vi "Main.vi"() -> ()   [LabVIEW 2018]
doc: "This is the main VI for the application using the VICI universal electric actuator.\n\n\n(Nimble Focus Consulting 2019)"
uses:
  controls/Timing and Position Entry.ctl
  controls/Application States.ctl
  subVIs/Elapsed Timer FGV/Enum - Programme Checker Machine State Typedef.ctl
panel:
  out "Current Actuation Cycles":u32
  in  "Get Current No. of Cycles":bool
  out "Current Time (s)":u32
  out "Current Position":u32
  in  "Manual Control Tab":enum32{"Page 1"}(tab)
  in  "Set Position":bool
  in  "Decrement Position":bool
  in  "Increment Position":bool
  in  "Home":bool
  in  "Get Position":bool
  out "Current Position":u32
  in  "New Position":u32=1 min=1 max=100
  in  "Start":bool
  out "No. of entries":i32
  out "Current Entry":T1
  in  "Abort":bool
  in  "Exit":bool
  in  "Clear List":bool
  in  "Timing and Position List":T1[](array[typedef])
  in  "VISA resource name":refnum<visa-resource-name>
  # "Operation Information"
  # "For program use - do not remove."
  # "Actuator Manual Controls"
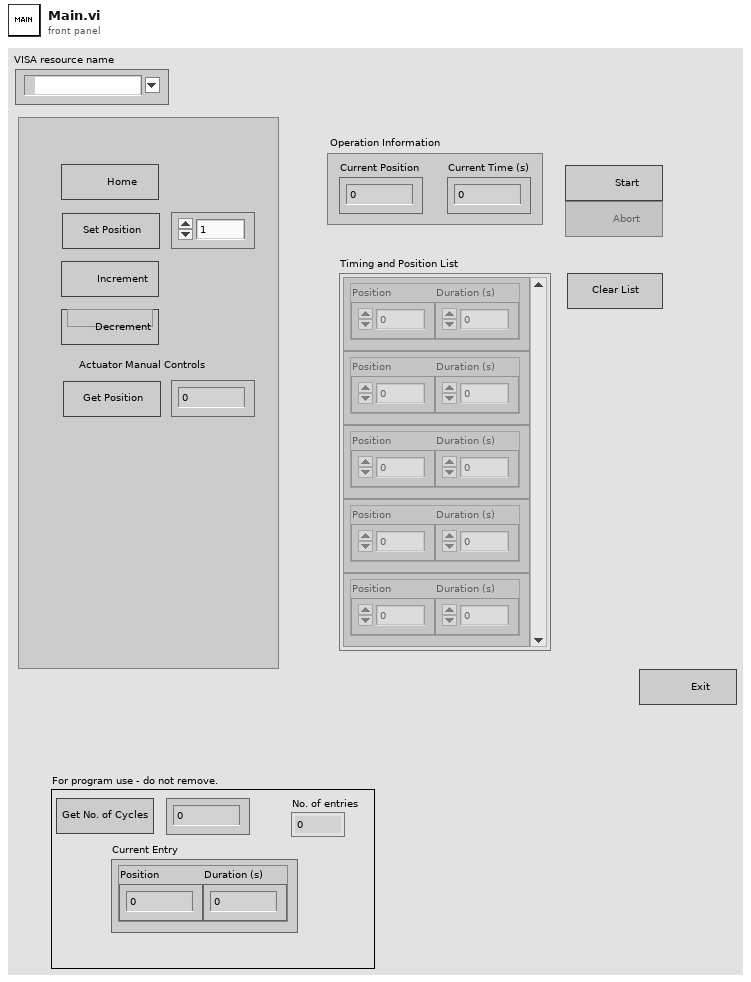
[diagram p1: front panel]
types:
  T1 = typedef "Timing and Position Entry.ctl" = cluster{"Position":u32, "Duration (s)":i32}
  T2 = typedef "Application States.ctl" = enum16{"Initialize", "Wait for Event", "Set Position", "Get Current Position", "Get Current No. of Cycles", "Home Actuator", "Increment Position", "Decrement Position", "Start Operation", "Retrieve Next Entry", "Set Position and Reset Timing", "Check Elapsed Time", "End Operation", "No More Entries Dialog", "Exit"}
  T3 = enum8{"Enabled", "Disabled", "Disabled and Grayed Out"}
  T4 = typedef "Enum - Programme Checker Machine State Typedef.ctl" = enum16{"Reset", "Check Elapsed Time"}
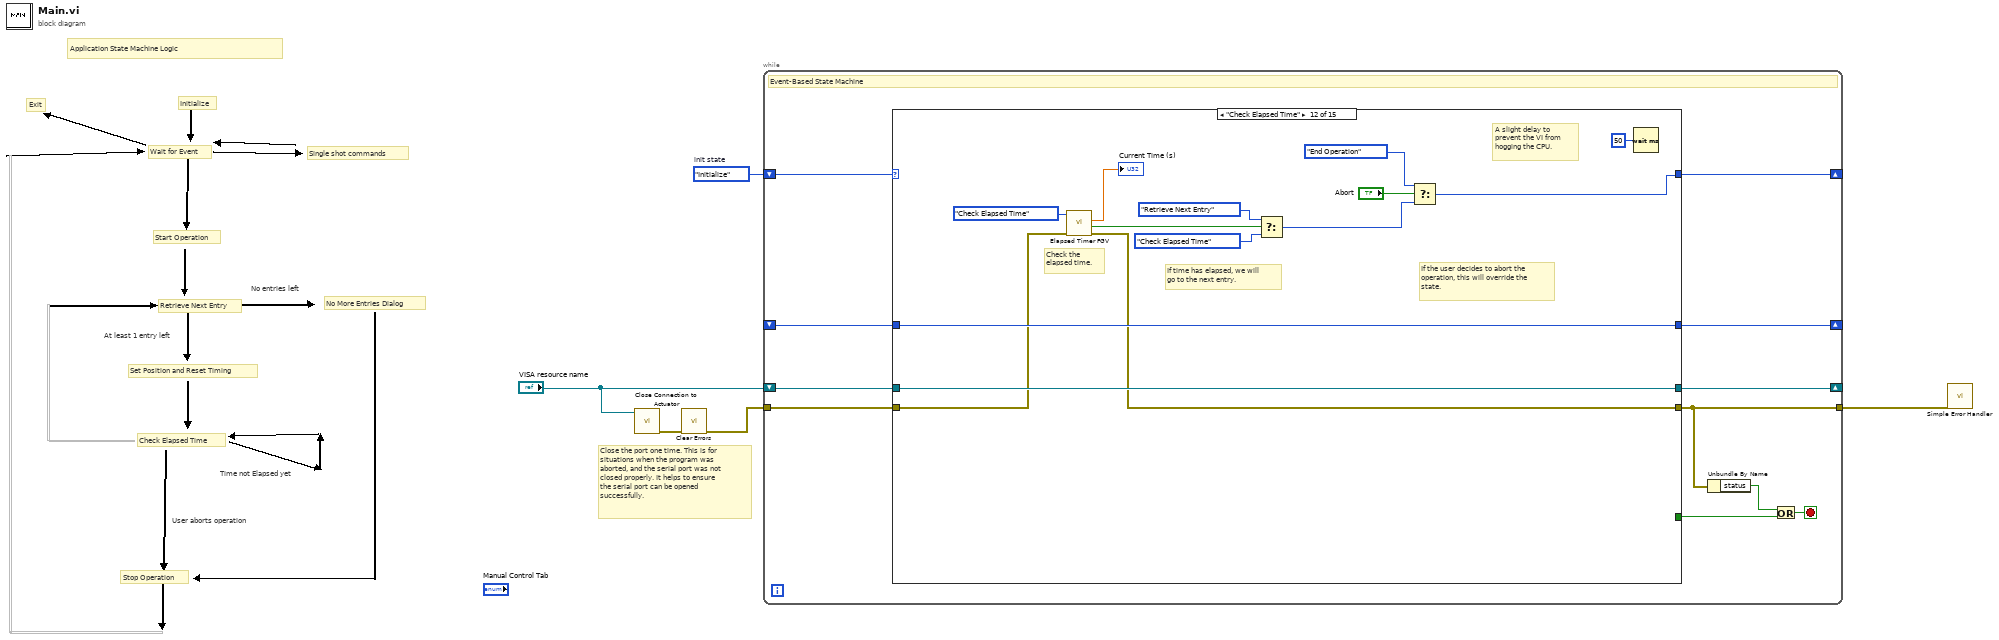
[diagram p0: block diagram]
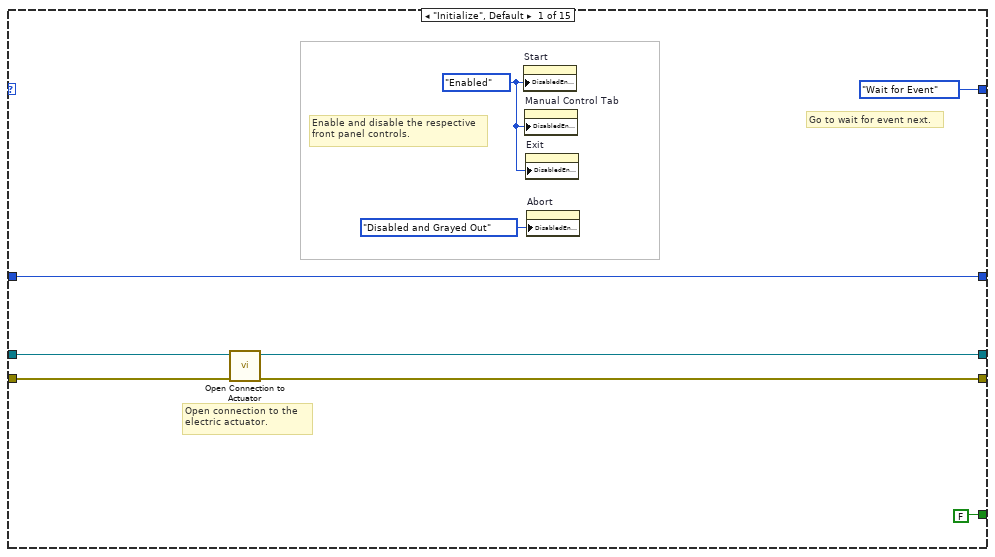
[diagram p2: hidden frame]
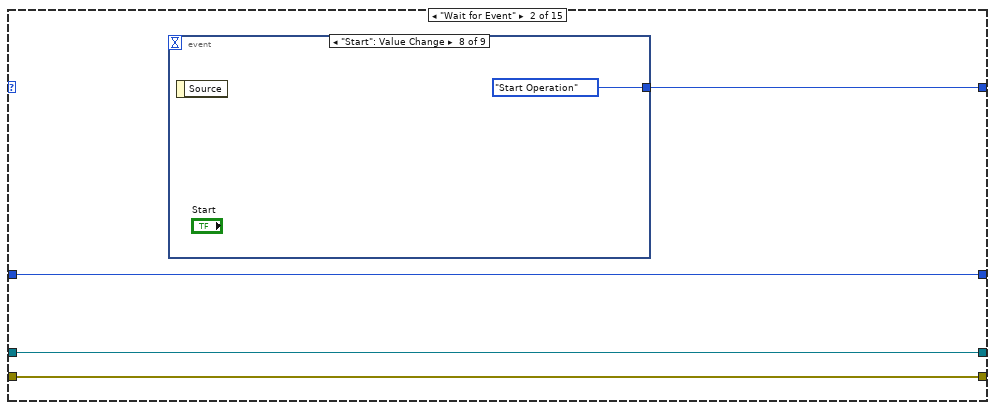
[diagram p3: hidden frame]
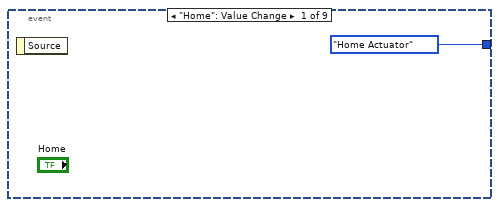
[diagram p4: hidden frame]
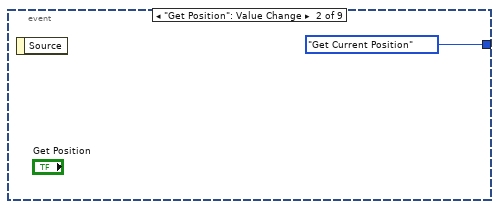
[diagram p5: hidden frame]
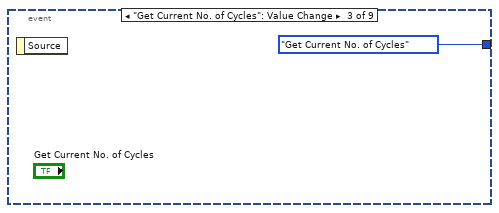
[diagram p6: hidden frame]
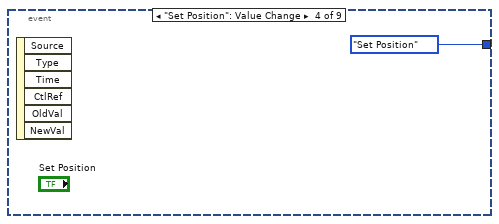
[diagram p7: hidden frame]
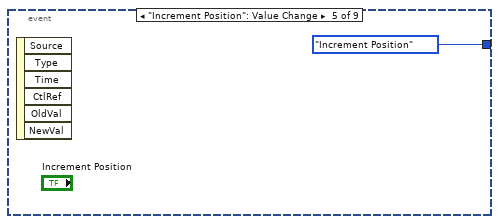
[diagram p8: hidden frame]
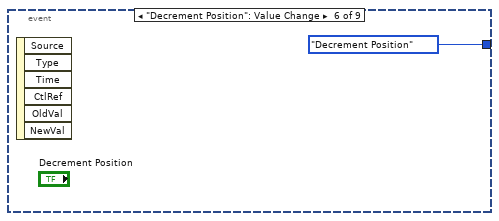
[diagram p9: hidden frame]
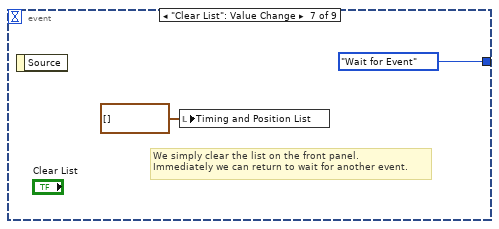
[diagram p10: hidden frame]
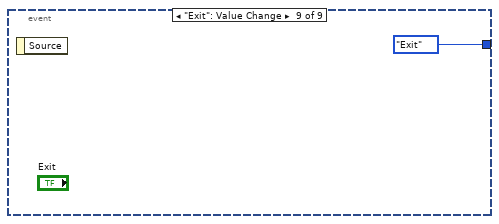
[diagram p11: hidden frame]
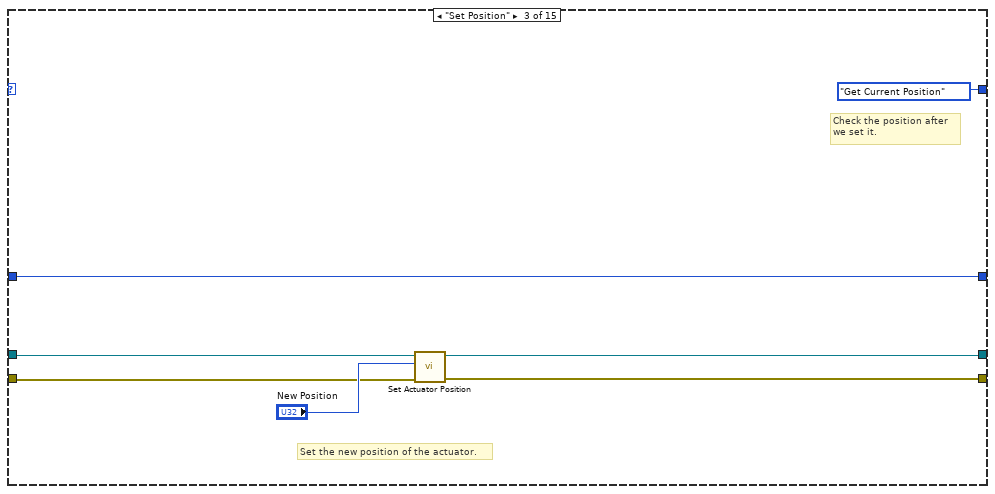
[diagram p12: hidden frame]
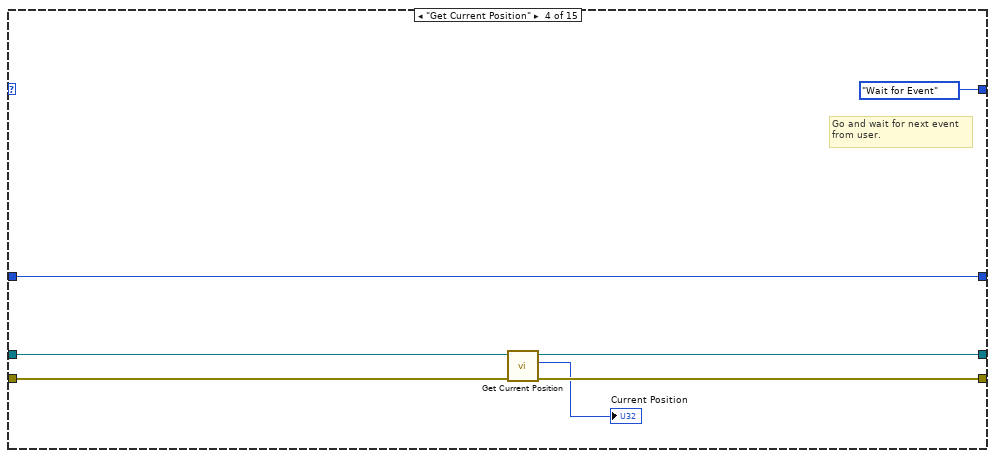
[diagram p13: hidden frame]
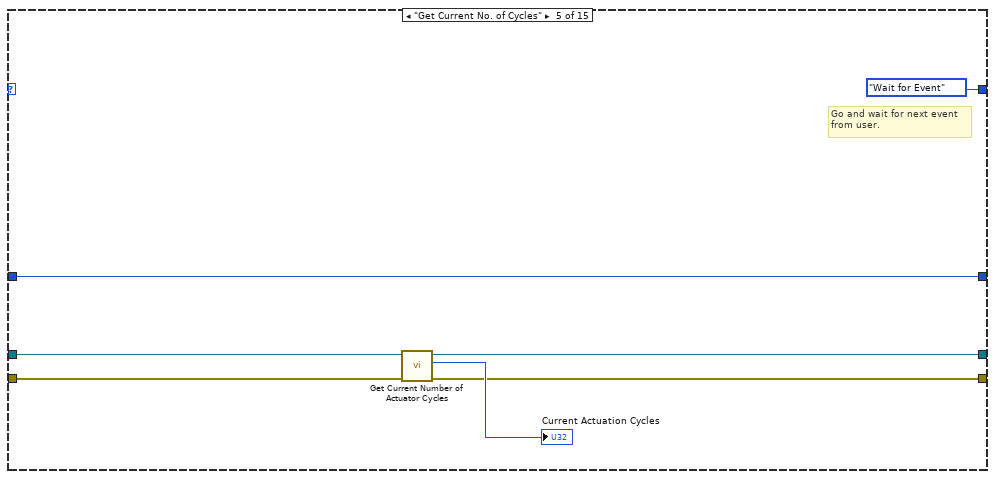
[diagram p14: hidden frame]
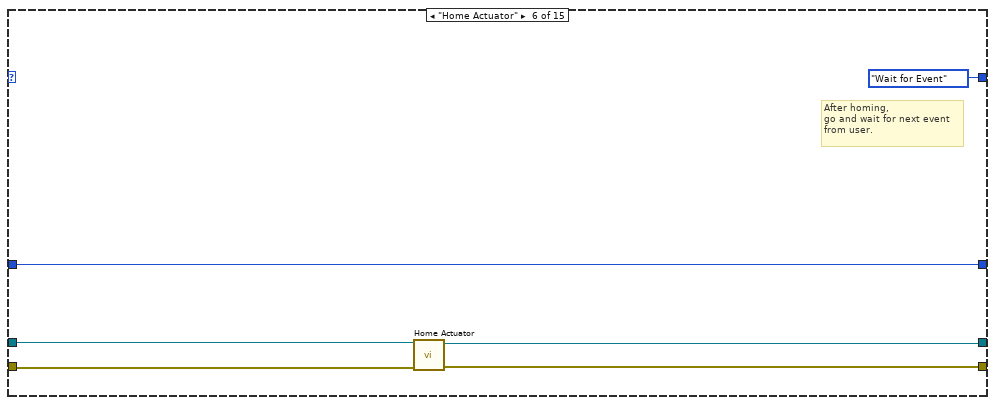
[diagram p15: hidden frame]
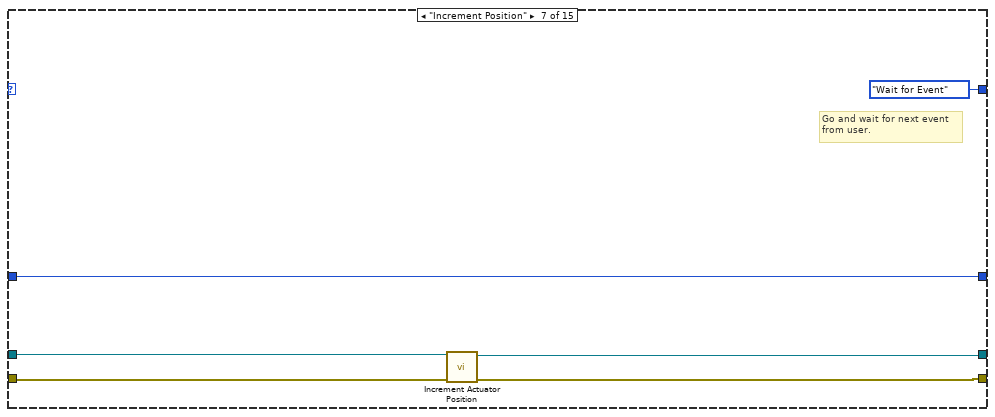
[diagram p16: hidden frame]
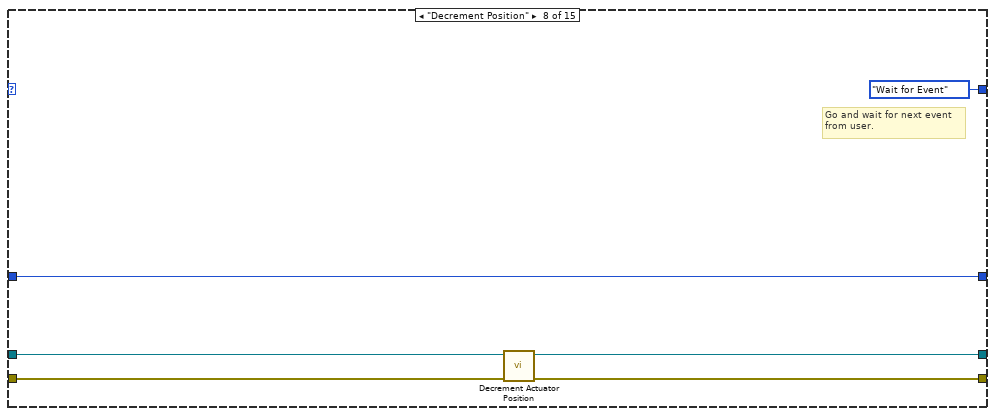
[diagram p17: hidden frame]
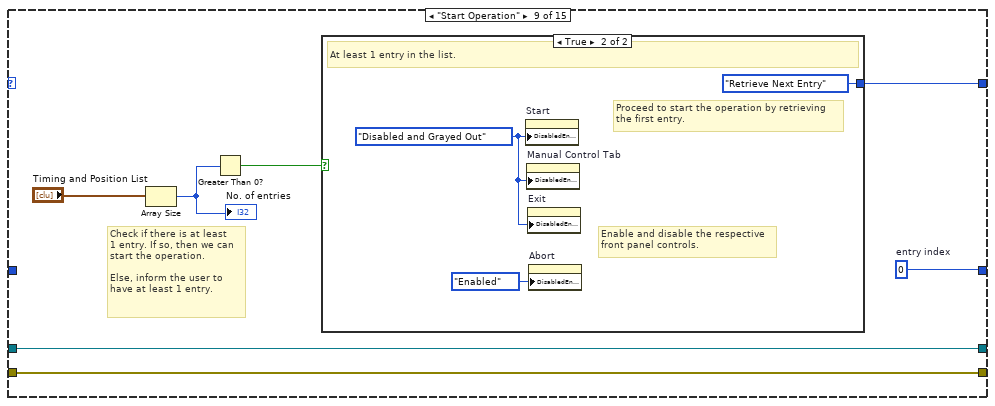
[diagram p18: hidden frame]
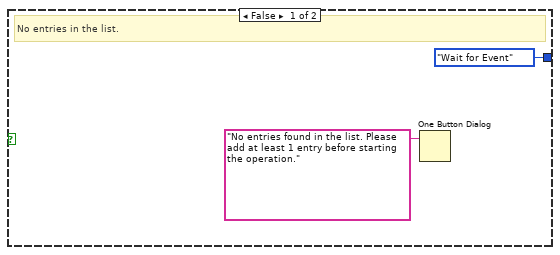
[diagram p19: hidden frame]
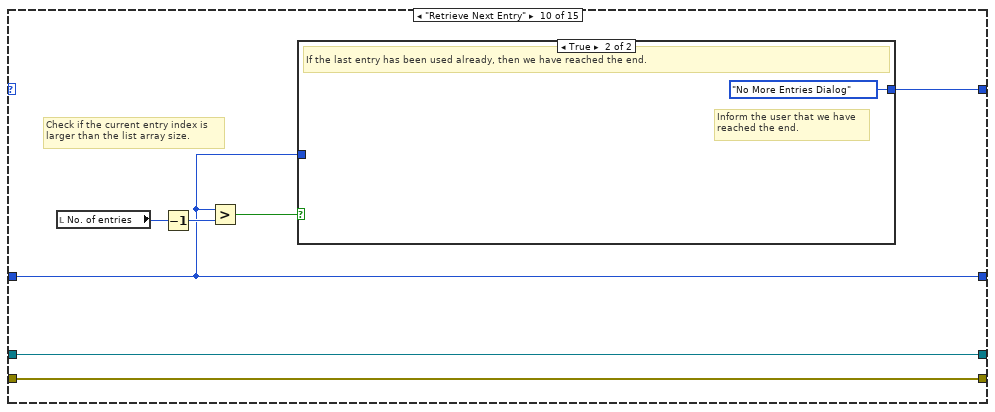
[diagram p20: hidden frame]
diagram:
  w5 = Application_States."Initialize"  # init state
  # "Application State Machine Logic"
  # "Exit"
  # "Close the port one time. This is for\nsituations when the program was\naborted, and the serial port was not\nclosed properly. It helps to ensure\nthe serial port can be opened\nsuccessfully."
  # "Stop Operation"
  # "User aborts operation"
  # "Time not Elapsed yet"
  # "No More Entries Dialog"
  # "At least 1 entry left"
  # "No entries left"
  # "Check Elapsed Time"
  # "Set Position and Reset Timing"
  # "Retrieve Next Entry"
  # "Initialize"
  # "Single shot commands"
  # "Wait for Event"
  # "Start Operation"
  n1 = call "Close Connection to Actuator.vi"("VISA resource name"="VISA resource name") -> ("error out"=w3:errorcluster)  [unwired: 10 in]
  n2 = call <vilib>:"Clear Errors.vi"("error in (no error)"=w3) -> ("error out"=w1:errorcluster)  [unwired: 5 in, 1 out]
  n3 = while {
    tunnel: [w14] -> w4
    shift-right: [w15] -> _
    shift-left: "VISA resource name" -> [w10]
    shift-right: [w9] -> _
    shift-left: w5 -> [w16]
    tunnel: w1 -> [w8]
    shift-right: [w7] -> _
    shift-left: _ -> [w6]
    stop <- w12 stop-if-true
    # "Event-Based State Machine"
    n4 = case shown="\"Check Elapsed Time\"" w16 {
      tunnel: [w25 w28 w43 w49 w58 w64 w68 w73 w80 w92 w105 w126 w130 w136 refnum<visa-resource-name> refnum ("VISA resource name")] -> w15
      tunnel: [w24 w27 w42 w48 w56 w63 w69 w74 w79 w91 w110 w119 w129 w135 w143] -> w14
      tunnel: [FALSE _ _ _ _ _ _ _ _ _ _ _ _ _ TRUE] -> w11
      tunnel: w10 -> [w21 w28 w44 w51 w59 w65 w71 w76 w80 w92 w108 w126 w130 w136 w145]
      tunnel: [Application_States."Wait for Event" ("init state") w29 Application_States."Get Current Position" ("init state") Application_States."Wait for Event" ("init state") Application_States."Wait for Event" ("init state") Application_States."Wait for Event" ("init state") Application_States."Wait for Event" ("init state") Application_States."Wait for Event" ("init state") w82 w94 Application_States."Check Elapsed Time" ("init state") w115 Application_States."Wait for Event" ("init state") Application_States."End Operation" ("init state") Application_States."Exit" ("init state")] -> w9
      tunnel: w8 -> [w20 w27 w41 w50 w55 w62 w70 w75 w79 w91 w107 w120 w129 w135 w144]
      tunnel: [w19 w26 w40 w52 w54 w61 w67 w77 w81 w93 w103 w125 w131 w137 w141] -> w7
      tunnel: w6 -> [w19 w26 w40 w52 w54 w61 w67 w77 _ w93 w109 w125 w131 w137 w141]
      frame "Initialize", Default {
        w17 = T3."Enabled" ("Disabled")
        # "Enable and disable the respective\nfront panel controls."
        # "Go to wait for event next."
        # "Open connection to the\nelectric actuator."
        n5 = call "Open Connection to Actuator.vi"("error in (no error)"=w20, "VISA resource name"=w21) -> ("error out"=w24:errorcluster, "VISA resource name out"=w25:refnum<visa-resource-name>)  [unwired: 8 in]
        n6 = property on="Start" class="Bool"("DisabledEnum"=w17) -> ()  [unwired: 2 in, 2 out]
        n7 = property on="Manual Control Tab" class="TabCtl (strict)"("DisabledEnum"=w17) -> ()  [unwired: 2 in, 2 out]
        n8 = property on="Exit" class="Bool"("DisabledEnum"=w17) -> ()  [unwired: 2 in, 2 out]
        n9 = property on="Abort" class="Bool"("DisabledEnum"=T3."Disabled and Grayed Out" ("Disabled")) -> ()  [unwired: 2 in, 2 out]
      }
      frame "Wait for Event" {
        n10 = event shown="[7] \"Start\": Value Change" {
          selector: _ -> [_ _ _ _ _ _ _ _ _]
          dyn-events: _ -> [_ _ _ _ _ _ _ _ _]
          timeout: _ -> [_ _ _ _ _ _ _ _ _]
          tunnel: [Application_States."Home Actuator" ("init state") Application_States."Get Current Position" ("init state") Application_States."Get Current No. of Cycles" ("init state") Application_States."Set Position" ("init state") Application_States."Increment Position" ("init state") Application_States."Decrement Position" ("init state") Application_States."Wait for Event" ("init state") Application_States."Start Operation" ("init state") Application_States."Exit" ("init state")] -> w29
          event "Home": Value Change {
            n11 = event-data() -> ()  [unwired: 1 in, 1 out]
          }
          event "Get Position": Value Change {
            n12 = event-data() -> ()  [unwired: 1 in, 1 out]
          }
          event "Get Current No. of Cycles": Value Change {
            n13 = event-data() -> ()  [unwired: 1 in, 1 out]
          }
          event "Set Position": Value Change {
            n14 = event-data() -> ()  [unwired: 1 in, 6 out]
          }
          event "Increment Position": Value Change {
            n15 = event-data() -> ()  [unwired: 1 in, 6 out]
          }
          event "Decrement Position": Value Change {
            n16 = event-data() -> ()  [unwired: 1 in, 6 out]
          }
          event "Clear List": Value Change {
            # "We simply clear the list on the front panel.\nImmediately we can return to wait for another event."
            n17 = event-data() -> ()  [unwired: 1 in, 1 out]
            n18 = local write "Timing and Position List"(T1[] [] ("Timing and Position List")) -> ()
          }
          event "Start": Value Change {
            n19 = event-data() -> ()  [unwired: 1 in, 1 out]
          }
          event "Exit": Value Change {
            n20 = event-data() -> ()  [unwired: 1 in, 1 out]
          }
        }
      }
      frame "Set Position" {
        # "Check the position after\nwe set it."
        # "Set the new position of the actuator."
        n21 = call "Set Actuator Position.vi"("error in (no error)"=w41, "Position (1 to NP)"="New Position", "VISA resource name"=w44) -> ("error out"=w42:errorcluster, "VISA resource name out"=w43:refnum<visa-resource-name>)  [unwired: 7 in]
      }
      frame "Get Current Position" {
        # "Go and wait for next event\nfrom user."
        n22 = call "Get Current Position.vi"("error in (no error)"=w50, "VISA resource name"=w51) -> ("error out"=w48:errorcluster, "Current Position out"=→"Current Position":u32, "VISA resource name out"=w49:refnum<visa-resource-name>)  [unwired: 7 in]
      }
      frame "Get Current No. of Cycles" {
        # "Go and wait for next event\nfrom user."
        n23 = call "Get Current Number of Actuator Cycles.vi"("error in (no error)"=w55, "VISA resource name"=w59) -> ("error out"=w56:errorcluster, "Current Number of Actuation Cycles out"=→"Current Actuation Cycles":u32, "VISA resource name out"=w58:refnum<visa-resource-name>)  [unwired: 7 in]
      }
      frame "Home Actuator" {
        # "After homing, \ngo and wait for next event\nfrom user."
        n24 = call "Home Actuator.vi"("error in (no error)"=w62, "VISA resource name"=w65) -> ("error out"=w63:errorcluster, "VISA resource name out"=w64:refnum<visa-resource-name>)  [unwired: 8 in]
      }
      frame "Increment Position" {
        # "Go and wait for next event\nfrom user."
        n25 = call "Increment Actuator Position.vi"("error in (no error)"=w70, "VISA resource name"=w71) -> ("error out"=w69:errorcluster, "VISA resource name out"=w68:refnum<visa-resource-name>)  [unwired: 8 in]
      }
      frame "Decrement Position" {
        # "Go and wait for next event\nfrom user."
        n26 = call "Decrement Actuator Position.vi"("error in (no error)"=w75, "VISA resource name"=w76) -> ("error out"=w74:errorcluster, "VISA resource name out"=w73:refnum<visa-resource-name>)  [unwired: 8 in]
      }
      frame "Start Operation" {
        w81 = 0  # entry index
        # "Check if there is at least\n1 entry. If so, then we can\nstart the operation.\n\nElse, inform the user to\nhave at least 1 entry."
        n27 = Array Size(array="Timing and Position List") -> (size(s)=w84:i32)
        "No. of entries" <- w84
        n28 = Greater Than 0?(x=w84) -> (x > 0?=w83:bool)
        n29 = case shown="True" w83 {
          tunnel: [Application_States."Wait for Event" ("init state") Application_States."Retrieve Next Entry" ("init state")] -> w82
          frame False {
            # "No entries in the list."
            n30 = One Button Dialog(message="No entries found in the list. Please add at least 1 entry before starting the operation.") -> ()  [unwired: 1 in, 1 out]
          }
          frame True {
            w88 = T3."Disabled and Grayed Out" ("Disabled")
            # "Enable and disable the respective\nfront panel controls."
            # "Proceed to start the operation by retrieving\nthe first entry."
            # "At least 1 entry in the list."
            n31 = property on="Start" class="Bool"("DisabledEnum"=w88) -> ()  [unwired: 2 in, 2 out]
            n32 = property on="Manual Control Tab" class="TabCtl (strict)"("DisabledEnum"=w88) -> ()  [unwired: 2 in, 2 out]
            n33 = property on="Exit" class="Bool"("DisabledEnum"=w88) -> ()  [unwired: 2 in, 2 out]
            n34 = property on="Abort" class="Bool"("DisabledEnum"=T3."Enabled" ("Disabled")) -> ()  [unwired: 2 in, 2 out]
          }
        }
      }
      frame "Retrieve Next Entry" {
        # "Check if the current entry index is\nlarger than the list array size."
        n35 = local read "No. of entries"() -> (w96:i32)
        n36 = Decrement(x=w96) -> (x-1=w97:i32)
        n37 = Greater?(x=w93, y=w97) -> (0:w95:bool)
        n38 = case shown="True" w95 {
          tunnel: [Application_States."Set Position and Reset Timing" ("init state") Application_States."No More Entries Dialog" ("init state")] -> w94
          tunnel: w93 -> [w100 _]
          frame False {
            # "Proceed to set the position and\nreset timing."
            # "If there is still at least 1 unused entry, then we will extract it."
            n39 = local read "Timing and Position List"() -> (w101:T1[])
            n40 = Index Array(array=w101, index=w100) -> (element=→"Current Entry":T1)
          }
          frame True {
            # "Inform the user that we have\nreached the end."
            # "If the last entry has been used already, then we have reached the end."
          }
        }
      }
      frame "Set Position and Reset Timing" {
        # "Increment the current entry index"
        # "Then proceed to check\nthe elapsed time."
        # "Reset the elapsed timer."
        # "Set the new position...."
        n41 = local read "Current Entry"() -> (w114:T1)
        n42 = Unbundle By Name(w114) -> ("Duration (s)"=w111:i32, "Position"=w104:u32)
        "Current Position" <- w104
        n43 = call "Set Actuator Position.vi"("error in (no error)"=w107, "Position (1 to NP)"=w104, "VISA resource name"=w108) -> ("error out"=w106:errorcluster, "VISA resource name out"=w105:refnum<visa-resource-name>)  [unwired: 7 in]
        n44 = Increment(x=w109) -> (x+1=w103:i32)
        n45 = call "Elapsed Timer FGV.vi"("error in (no error)"=w106, "Time to count down to (s)"=w111, "Command"=Enum_-_Programme_Checker_Machine_State_Typedef."Reset") -> ("error out"=w110:errorcluster)  [unwired: 6 in, 2 out]
      }
      frame "Check Elapsed Time" {
        # "A slight delay to\nprevent the VI from\nhogging the CPU."
        # "If the user decides to abort the\noperation, this will override the\nstate."
        # "If time has elapsed, we will\ngo to the next entry."
        # "Check the\nelapsed time."
        n46 = call "Elapsed Timer FGV.vi"("error in (no error)"=w120, "Command"=Enum_-_Programme_Checker_Machine_State_Typedef."Check Elapsed Time") -> ("error out"=w119:errorcluster, "Elapsed?"=w123:bool, "Current Elapsed time (s)"=→"Current Time (s)":dbl)  [unwired: 7 in]
        n47 = Select(t=Application_States."Retrieve Next Entry" ("init state"), s=w123, f=Application_States."Check Elapsed Time" ("init state")) -> (s? t:f=w117:T2)
        n48 = Select(t=Application_States."End Operation", s="Abort", f=w117) -> (s? t:f=w115:T2)
        n49 = Wait (ms)(milliseconds to wait=u32 50) -> ()  [unwired: 1 out]
      }
      frame "End Operation" {
        w132 = T3."Enabled" ("Disabled")
        # "Enable and disable the respective\nfront panel controls."
        n50 = property on="Start" class="Bool"("DisabledEnum"=w132) -> ()  [unwired: 2 in, 2 out]
        n51 = property on="Manual Control Tab" class="TabCtl (strict)"("DisabledEnum"=w132) -> ()  [unwired: 2 in, 2 out]
        n52 = property on="Exit" class="Bool"("DisabledEnum"=w132) -> ()  [unwired: 2 in, 2 out]
        n53 = property on="Abort" class="Bool"("DisabledEnum"=T3."Disabled and Grayed Out" ("Disabled")) -> ()  [unwired: 2 in, 2 out]
      }
      frame "No More Entries Dialog" {
        # "Proceed to end operation."
        n54 = One Button Dialog(message="No more entries left. The operation will now stop.") -> ()  [unwired: 1 in, 1 out]
      }
      frame "Exit" {
        # "Close connection to the actuator."
        n55 = call "Close Connection to Actuator.vi"("error in (no error)"=w144, "VISA resource name"=w145) -> ("error out"=w143:errorcluster)  [unwired: 9 in]
      }
    }
    n56 = Unbundle By Name(w14) -> ("status"=w13:bool)
    n57 = Or(x=w13, y=w11) -> (x .or. y?=w12:bool)
  }
  n58 = call <vilib>:"Simple Error Handler.vi"("error in (no error)"=w4) -> ()  [unwired: 4 in, 5 out]
